vi "Top VI FG.vi"(7 "Set (F)":bool, 10 "error in (no error)":errorcluster, 11 "Top-Level VI In":refnum<vi>) -> (2 "error out":errorcluster, 3 "Top-Level VI":refnum<vi>)   [LabVIEW 2020, in "PicoG-App.lvlib"]
uses:
  PicoG-App.lvlib
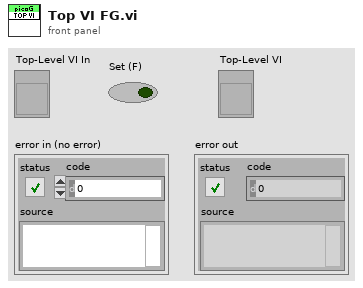
[diagram p1: front panel]
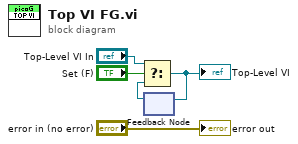
[diagram p0: block diagram]
diagram:
  n1 = feedback #1() -> (w1:refnum<vi>)  [unwired: 1 in]
  n2 = Select(t="Top-Level VI In", s="Set (F)", f=w1) -> (s? t:f=w2:refnum<vi>)
  "Top-Level VI" <- w2
  n3 = feedback-in #1(w2) -> ()
  "error out" <- "error in (no error)"
